vi "Frequency Modulator Dynamic.vi"(10 "Frequency":dbl=1000.0, 11 "Sine":dynamicdata(waveform)) -> (3 "Dynamic Data":dynamicdata(waveform))   [LabVIEW 2014, in "Aquisicao de Dados.lvlib"]
uses:
  Aquisicao de Dados.lvlib
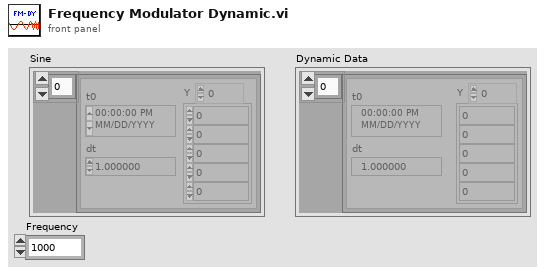
[diagram p1: front panel]
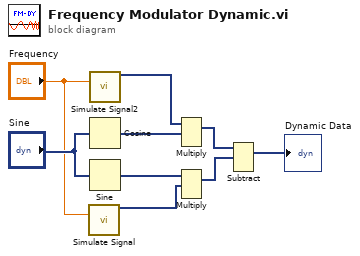
[diagram p0: block diagram]
diagram:
  n1 = call "Simulate Signal"("Frequency"="Frequency") -> ("Sine"=w7:dynamicdata)  [unwired: 13 in, 1 out]
  n2 = call "Simulate Signal2"("Frequency"="Frequency") -> ("Sine"=w6:dynamicdata)  [unwired: 13 in, 1 out]
  n3 = Cosine(x="Sine") -> (cos(x)=w2:dynamicdata)
  n4 = Sine(x="Sine") -> (sin(x)=w3:dynamicdata)
  n5 = Multiply(1:w2, 2:w6) -> (0:w4:dynamicdata)  [unwired: 1 in, 1 out]
  n6 = Multiply(1:w7, 2:w3) -> (0:w5:dynamicdata)  [unwired: 1 in, 1 out]
  n7 = Subtract(1:w5, 2:w4) -> (0:→"Dynamic Data":dynamicdata)  [unwired: 1 in, 1 out]
